vi "DAQNavi Read (Counter 1D Count Value 1Chan NSamp).vi"(8 "error in (no error)":errorcluster, 9 "number of samples per channel to read":u32=10, 10 "timeout":dbl=10.0, 11 "task in":i32) -> (0 "error out":errorcluster, 2 "data":i32[](array[numeric]), 3 "task out":i32)   [LabVIEW 2020]
uses:
  DAQNavi_LV.dll
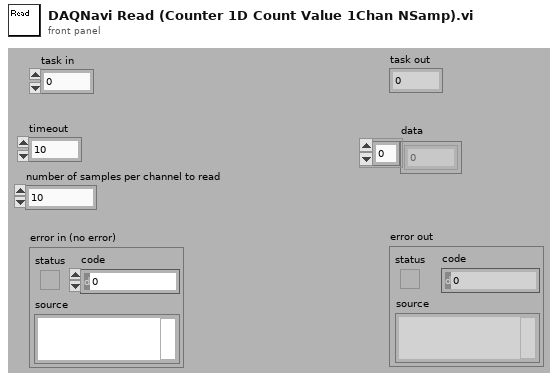
[diagram p1: front panel]
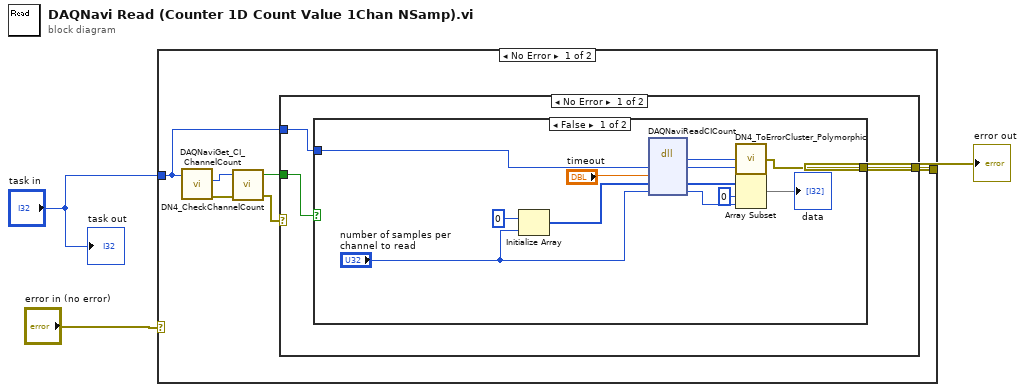
[diagram p0: block diagram]
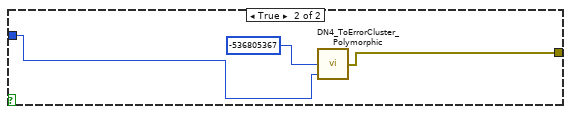
[diagram p2: hidden frame]
diagram:
  n1 = case shown="No Error" "error in (no error)" {
    selector: "error in (no error)" -> [_ w29]
    tunnel: "task in" -> [w5 _]
    tunnel: [w9 w29] -> w1
    frame No Error {
      n2 = call "DAQNaviGet_CI_ChannelCount.vi"("task in"=w5) -> ("error out"=w8:errorcluster, "channel count"=w4:i32)  [unwired: 1 in, 8 out]
      n3 = call "DN4_CheckChannelCount.vi"("error out"=w8, "channel count"=w4) -> ("error IO"=w7:errorcluster, "greater than 1?"=w6:bool)  [unwired: 2 out]
      n4 = case shown="No Error" w7 {
        selector: w7 -> [_ w28]
        tunnel: [w12 w28] -> w9
        tunnel: w6 -> [w11 _]
        tunnel: w5 -> [w10 _]
        frame No Error {
          n5 = case shown="False" w11 {
            tunnel: [w14 w25] -> w12
            tunnel: w10 -> [w13 w26]
            frame False {
              n6 = Initialize Array(0 ("element"), "number of samples per channel to read") -> (w16:i32[])
              n7 = dll-call lib="DAQNavi_LV.dll" fn="DAQNaviReadCICount"("taskID"=w13, "timeout"="timeout", "count"=w16, "samples"="number of samples per channel to read") -> ("return type"=w24:i32, "taskID"=w15:i32, "count"=w22:i32[], "samples"=w20:u32)  [unwired: 4 in, 2 out]
              n8 = call "DN4_ToErrorCluster_Polymorphic.vi"("task id"=w15, "error code"=w24) -> ("error out"=w14:errorcluster)  [unwired: 3 out]
              n9 = Array Subset(array=w22, index=0, length=w20) -> (→"data":i32[])
            }
            frame True {
              n10 = call "DN4_ToErrorCluster_Polymorphic.vi"("task id"=w26, "error code"=-536805367 ("error code (0)")) -> ("error out"=w25:errorcluster)  [unwired: 3 out]
            }
          }
        }
        frame Error {
        }
      }
    }
    frame Error {
    }
  }
  "error out" <- w1
  "task out" <- "task in"
